vi "AfterName.vi"(11 "The String":string) -> (3 "after \"Name\"":string)   [LabVIEW 2020]
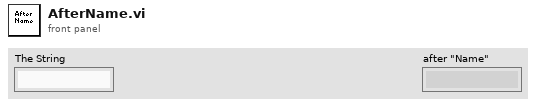
[diagram p1: front panel]
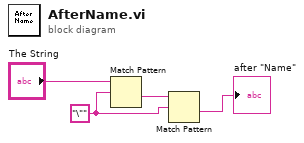
[diagram p0: block diagram]
diagram:
  w3 = "\"" ("regular expression")
  n1 = Match Pattern(string="The String", regular expression=w3) -> (after substring=w4:string)  [unwired: 1 in, 3 out]
  n2 = Match Pattern(string=w4, regular expression=w3) -> (after substring=→"after \"Name\"":string)  [unwired: 1 in, 3 out]
